vi "3446X_Reset.vi"(0 "User Reference":i32, 5 "error in (no error)":errorcluster) -> (19 "error out":errorcluster)   [LabVIEW 2015, in "3446X.lvclass"]
uses:
  3446X.lvclass
  DMM Virtual/DMM Virtual.lvclass
  <instrlib>/Agilent 3446X Series/Agilent 3446X Series.lvlib
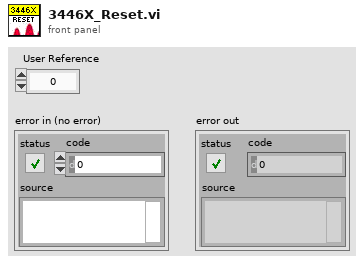
[diagram p1: front panel]
types:
  T1 = typedef "Class Attributes Cluster.ctl" = cluster{"Model Number":string, "Instrument Number":u8, "Rack ID":string, "Inst Mnemonic":string, "Comp Mnemonic":string, "Subsys Mnemonic":string, "IP Address":string, "Sub Address":string, "Firmware Rev":string, "Expected Options":string, "Required Options":string, "Excluded Options":string}
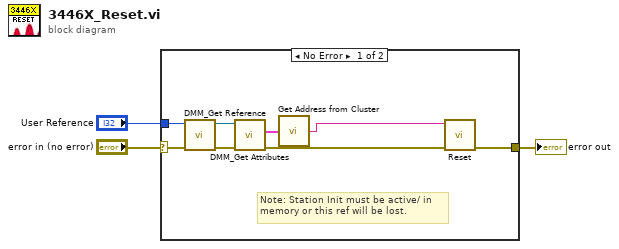
[diagram p0: block diagram]
diagram:
  n1 = case shown="No Error" "error in (no error)" {
    selector: "error in (no error)" -> [w11 w12]
    tunnel: [w6 w12] -> w2
    tunnel: "User Reference" -> [w8 _]
    frame No Error {
      # "Note: Station Init must be active/ in\nmemory or this ref will be lost."
      n2 = call "DMM_Get Reference.vi"("error in (no error)"=w11, "Instrument Reference"=w8) -> ("error out"=w10:errorcluster, "DMM Virtual.lvclass"=w9:refnum<class "DMM Virtual.lvclass">)  [unwired: 8 in]
      n3 = call-dynamic "DMM_Get Attributes.vi"("error in (no error)"=w10, "DMM Virtual in"=w9) -> ("error out"=w7:errorcluster, "Class Attributes"=w5:T1)  [unwired: 7 in, 1 out]
      n4 = call "Get Address from Cluster.vi"("Class Attributes"=w5) -> ("Address"=w4:string)  [unwired: 4 in]
      n5 = call <instrlib>:"Reset.vi"("error in (no error)"=w7, "VISA resource name"=w4) -> ("error out"=w6:errorcluster)  [unwired: 8 in, 1 out]
    }
    frame Error {
    }
  }
  "error out" <- w2
